vi "__SG_83630L_ONOFF.vi"(0 "ON/OFF":string="OFF", 2 "GPIB":string="19") -> ()   [LabVIEW 2017]
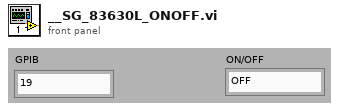
[diagram p1: front panel]
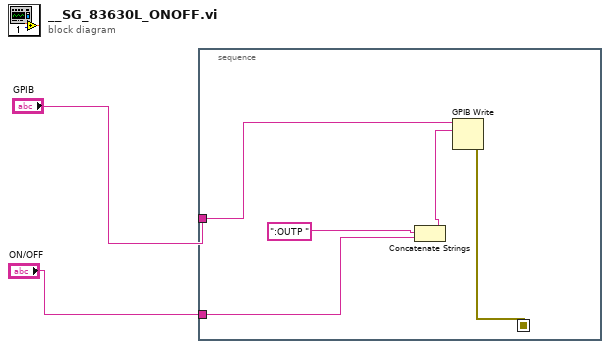
[diagram p0: block diagram]
diagram:
  n1 = stacked-sequence {
    seq-local: [w6] -> [_]
    tunnel: "GPIB" -> [w5]
    tunnel: "ON/OFF" -> [w3]
    frame #0 {
      n2 = Concatenate Strings(":OUTP ", w3) -> (w7:string)
      n3 = GPIB Write(0:w5, 1:w7) -> (6:w6:errorcluster)  [unwired: 3 in, 1 out]
    }
  }
